vi "Calc_Mode_Register_F4.vi"(8 "OSRS_Temp":T1, 9 "OSRS_Press":T1, 10 "PowerMode":T2=enum."Normal") -> (2 "F4_Register":u8=28 format="%08b")   [LabVIEW 2020, in "BMP208.lvclass"]
uses:
  BMP208.lvclass
  Controls/td_enum_powermode.ctl
  Controls/td_enum_osrsX.ctl
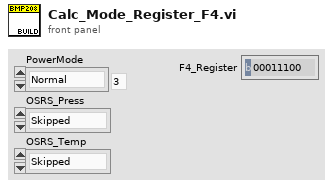
[diagram p1: front panel]
types:
  T1 = typedef "BMP208.lvclass/td_enum_osrsX.ctl" = enum16{"Skipped", "16b", "17b", "18b", "19b", "20b", "20b_2", "20b_3"}
  T2 = typedef "BMP208.lvclass/td_enum_powermode.ctl" = enum16{"Sleep", "Forced", "Forced_", "Normal"}
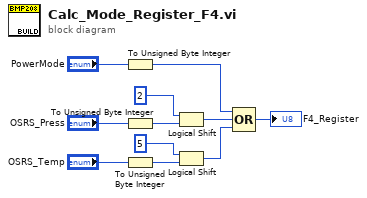
[diagram p0: block diagram]
diagram:
  n1 = To Unsigned Byte Integer(number="PowerMode") -> (unsigned 8bit integer=w5:u8)
  n2 = To Unsigned Byte Integer(number="OSRS_Press") -> (unsigned 8bit integer=w3:u8)
  n3 = To Unsigned Byte Integer(number="OSRS_Temp") -> (unsigned 8bit integer=w1:u8)
  n4 = Logical Shift(y=u8 2, x=w3) -> (x << y=w9:u8)
  n5 = Logical Shift(y=u8 5, x=w1) -> (x << y=w8:u8)
  n6 = Compound Arithmetic op=OR(w5, w9, w8) -> (→"F4_Register":u8)
